vi "S2C_CMD_Globals.vi"() -> ()   [LabVIEW 2015]
doc: "Globals for the Command Parameters panel."
panel:
  in  "Drivers":string[](array[string])
  in  "Command":string
  in  "Types":string[][][][](array[string])
  in  "Commands":string[][][][](array[string])
  in  "Active_Types":string[][][](array[string])
  in  "Active_Cmds":string[][][](array[string])
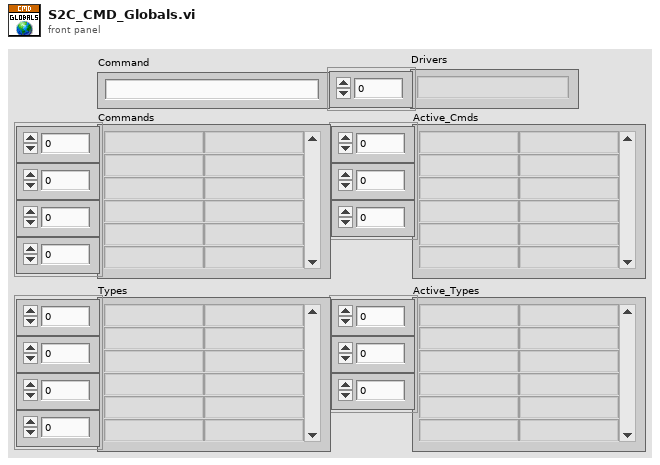
[diagram p1: front panel]
diagram:
